vi "SetParam.vi"(8 "error in (no error)":errorcluster caption="entrée d'erreur (pas d'erreur)", 10 "chi2_kernel":cluster{"gamma":dbl}={"gamma"=1.0}, 11 "Chi2_kernel.lvclass":refnum<class "Chi2_kernel.lvclass">) -> (0 "error out":errorcluster caption="sortie d'erreur", 3 "Chi2_kernel.lvclass":refnum<class "Chi2_kernel.lvclass">)   [LabVIEW 2020, in "Chi2_kernel.lvclass"]
doc: "Set Parameters"
uses:
  Chi2_kernel.lvclass
  Chi2_kernel.lvclass/Chi2_kernel.ctl
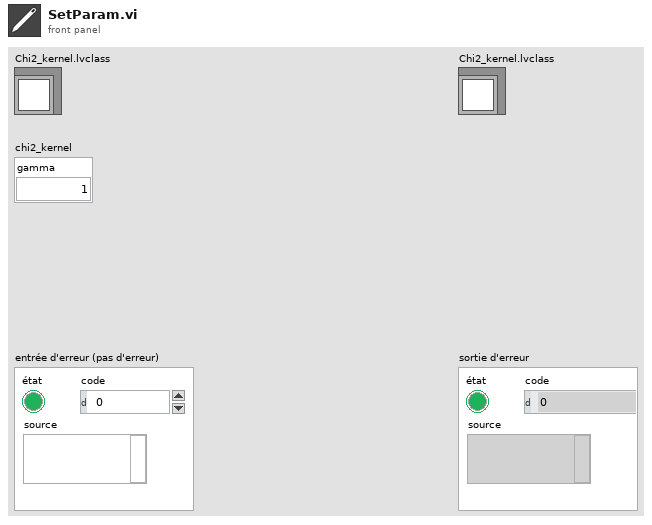
[diagram p1: front panel]
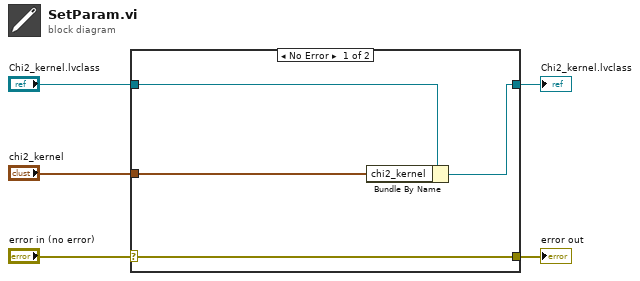
[diagram p0: block diagram]
diagram:
  n1 = case shown="No Error" "error in (no error)" {
    selector: "error in (no error)" -> [w9 w10]
    tunnel: [w9 w10] -> w4
    tunnel: [w7 w11] -> w2
    tunnel: "Chi2_kernel.lvclass" -> [w8 w11]
    tunnel: "chi2_kernel" -> [w6 _]
    frame No Error {
      n2 = Bundle By Name(cluster=w8, "chi2_kernel"=w6) -> (w7:refnum<class "Chi2_kernel.lvclass">)
    }
    frame Error {
    }
  }
  "error out" <- w4
  "Chi2_kernel.lvclass" <- w2
